vi "add_tag.vi"(8 "error in (no error)":errorcluster, 10 "tag":string, 11 "ImageCollection in":refnum<class "ImageCollection.lvclass">) -> (0 "error out":errorcluster, 3 "ImageCollection out":refnum<class "ImageCollection.lvclass">)   [LabVIEW 2010, in "ImageCollection.lvclass"]
uses:
  ImageCollection.lvclass
  ImageCollection.lvclass/ImageCollection.ctl
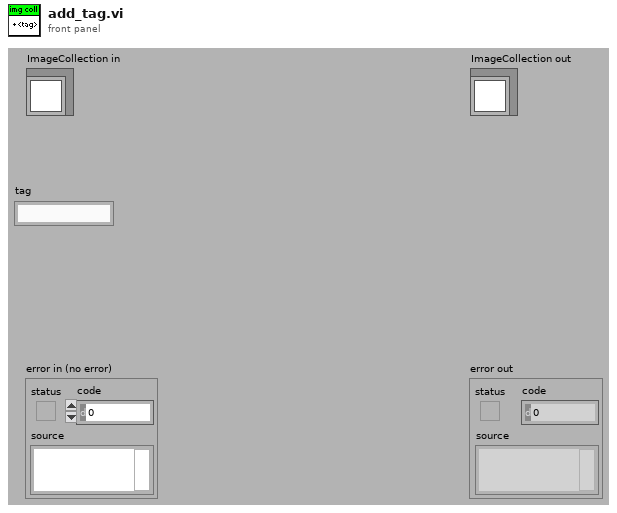
[diagram p1: front panel]
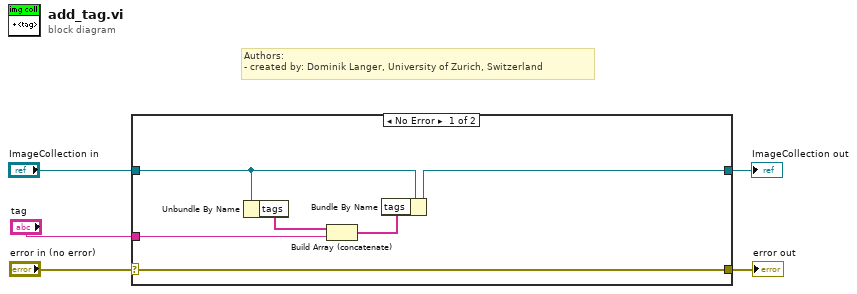
[diagram p0: block diagram]
diagram:
  # "Authors: \n- created by: Dominik Langer, University of Zurich, Switzerland"
  n1 = case shown="No Error" "error in (no error)" {
    selector: "error in (no error)" -> [w11 w13]
    tunnel: [w11 w13] -> w4
    tunnel: [w9 w12] -> w2
    tunnel: "ImageCollection in" -> [w10 w12]
    tunnel: "tag" -> [w6 _]
    frame No Error {
      n2 = Unbundle By Name(w10) -> ("tags"=w8:string[])
      n3 = Build Array (concatenate)(w8, w6) -> (w7:string[])
      n4 = Bundle By Name(cluster=w10, "tags"=w7) -> (w9:refnum<class "ImageCollection.lvclass">)
    }
    frame Error {
    }
  }
  "error out" <- w4
  "ImageCollection out" <- w2
